vi "Instrument_Setting.vi"(8 "错误输入（无错误）":errorcluster, 9 "id":string[](array[string]), 10 "Get_USB_Resouce":string[](array[string]), 11 "Address Cluster":T1={"SPU"=refnum, "MPM"=[], "Port_Count"=0.0, "MPM_Count"=0.0, "SPU_Resource"=[], "USB_Resource"=[], "MPM_Communicater"="", "MPM_Count"=0.0, "MPM_Address"=[], "MPM_Portnumber"=[], "SPU_DeviveID"="", "MPM_communcation_method"=[], "TSL_sweepstartwave"=0.0, "TSL_sweepstopwave"=0.0, "TSL_Address"="", "TSL_Communicater"="", "TSL"=refnum, "tsl_communcation_method"=3, "TSL_Portnumber"=0.0} {"tsl_communcation_method" items=["GPIB", "C232C", "TCPIP", "USB"]; "MPM_communcation_method" items=["GPIB", "C232C", "TCPIP", "USB"]}) -> (0 "错误输出":errorcluster, 2 "PowerMonitorType":enum16{"DAQ", "MPM_220", "TSL_LOGG"}(ring), 3 "Address Cluster out":T1={"SPU"=refnum, "MPM"=[], "Port_Count"=0.0, "MPM_Count"=0.0, "SPU_Resource"=[], "USB_Resource"=[], "MPM_Communicater"="", "MPM_Count"=0.0, "MPM_Address"=[], "MPM_Portnumber"=[], "SPU_DeviveID"="", "MPM_communcation_method"=[], "TSL_sweepstartwave"=0.0, "TSL_sweepstopwave"=0.0, "TSL_Address"="", "TSL_Communicater"="", "TSL"=refnum, "tsl_communcation_method"=3, "TSL_Portnumber"=0.0} {"tsl_communcation_method" items=["GPIB", "C232C", "TCPIP", "USB"]; "MPM_communcation_method" items=["GPIB", "C232C", "TCPIP", "USB"]})   [LabVIEW 2017]
doc: "Setting Form"
uses:
  CTL/Address Cluster.ctl
  D:/test/ILSTS/LV_IL/LV_IL_Sample_x86/DLL/InstrumentDLL.dll
  DLL/InstrumentDLL.dll
  Share/PowerMonitorType.vi
panel:
  in  "Product_MPM":enum32{"rdompm210", "rdompm220"}(radio) caption="Product"
  in  "Preformance":enum32{"rb_high_spec", "rb_standard"}(radio)
  out "Boolean":bool=TRUE
  in  "Port_Count":i32
  in  "btnconnect":bool
  in  "cmbSPU_dev":u16(ring) caption="Device"
  in  "IP Address_MPM 2":string caption="IP Address"
  in  "LAN Port_MPM 2":dbl caption="LAN Port"
  in  "GPIB Address_MPM 2":i32 caption="GPIB Address"
  in  "chkmulti_dev":bool
  in  "IP Address_MPM":string caption="IP Address"
  in  "LAN Port_MPM":dbl caption="LAN Port"
  in  "GPIB Address_MPM":i32=14 caption="GPIB Address"
  in  "Communication_MPM":enum32{"rdiGPIB_MPM", "rdiLAN_MPM"}(radio) caption="Communication"
  in  "IP Address_TSL":string caption="IP Address"
  in  "LAN Port_TSL":i32 caption="LAN Port"
  in  "GPIB Address_TSL":i32=1 caption="GPIB Address"
  in  "Usb resouce_TSL":u16(ring) caption="Usb resouce"
  in  "Communication_TSL":T2(radio) caption="Communication"
  in  "Product_TSL":enum32{"rdo550_TSL", "rdo570_TSL"}(radio) caption="Product"
  # "TSL"
  # "MPM"
  # "Device1"
  # "Device2"
  # "SPU"
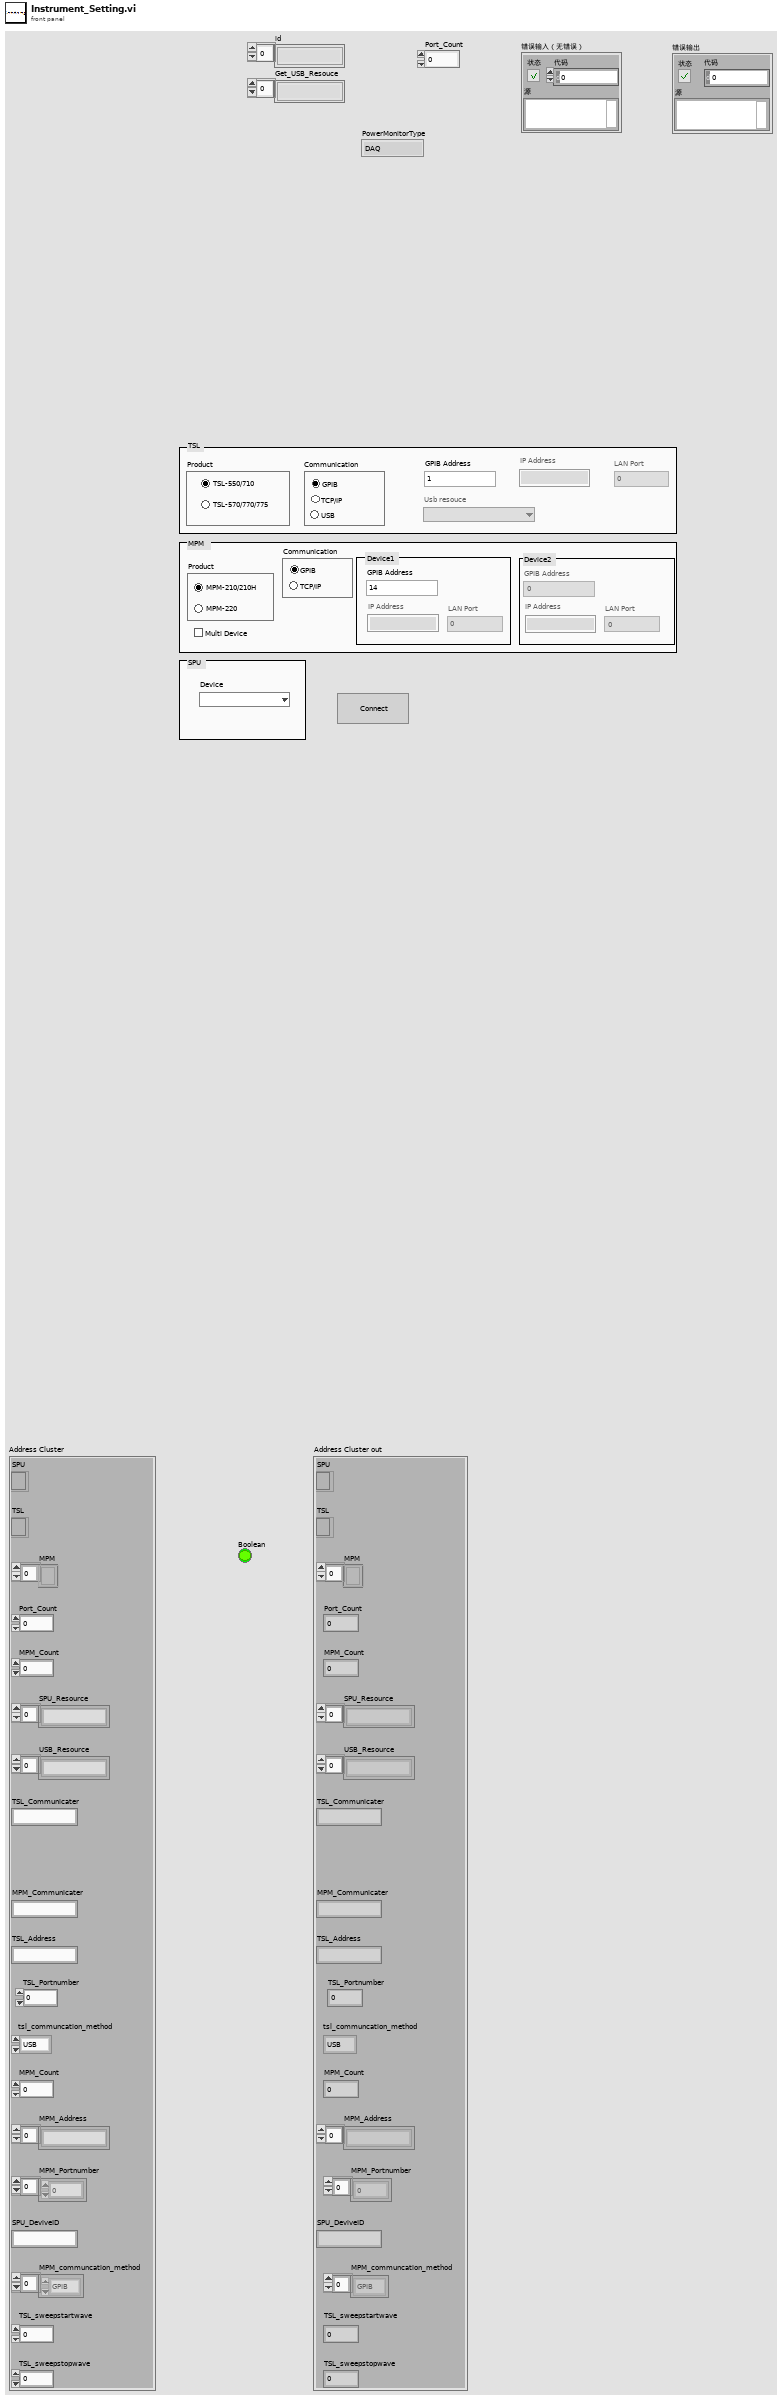
[diagram p1: front panel]
types:
  T1 = typedef "Address Cluster.ctl" = cluster{"SPU":refnum<k24>, "MPM":refnum<k24>[], "Port_Count":dbl, "MPM_Count":dbl, "SPU_Resource":string[], "USB_Resource":string[], "MPM_Communicater":string, "MPM_Count":dbl, "MPM_Address":string[], "MPM_Portnumber":dbl[], "SPU_DeviveID":string, "MPM_communcation_method":i32[], "TSL_sweepstartwave":dbl, "TSL_sweepstopwave":dbl, "TSL_Address":string, "TSL_Communicater":string, "TSL":refnum<k24>, "tsl_communcation_method":i32, "TSL_Portnumber":dbl}
  T2 = enum32{"rdiGPIB_TSL", "rdiLAN_TSL", "rdiUSB_TSL"}
  T3 = enum8{"Enabled", "Disabled", "Disabled and Grayed Out"}
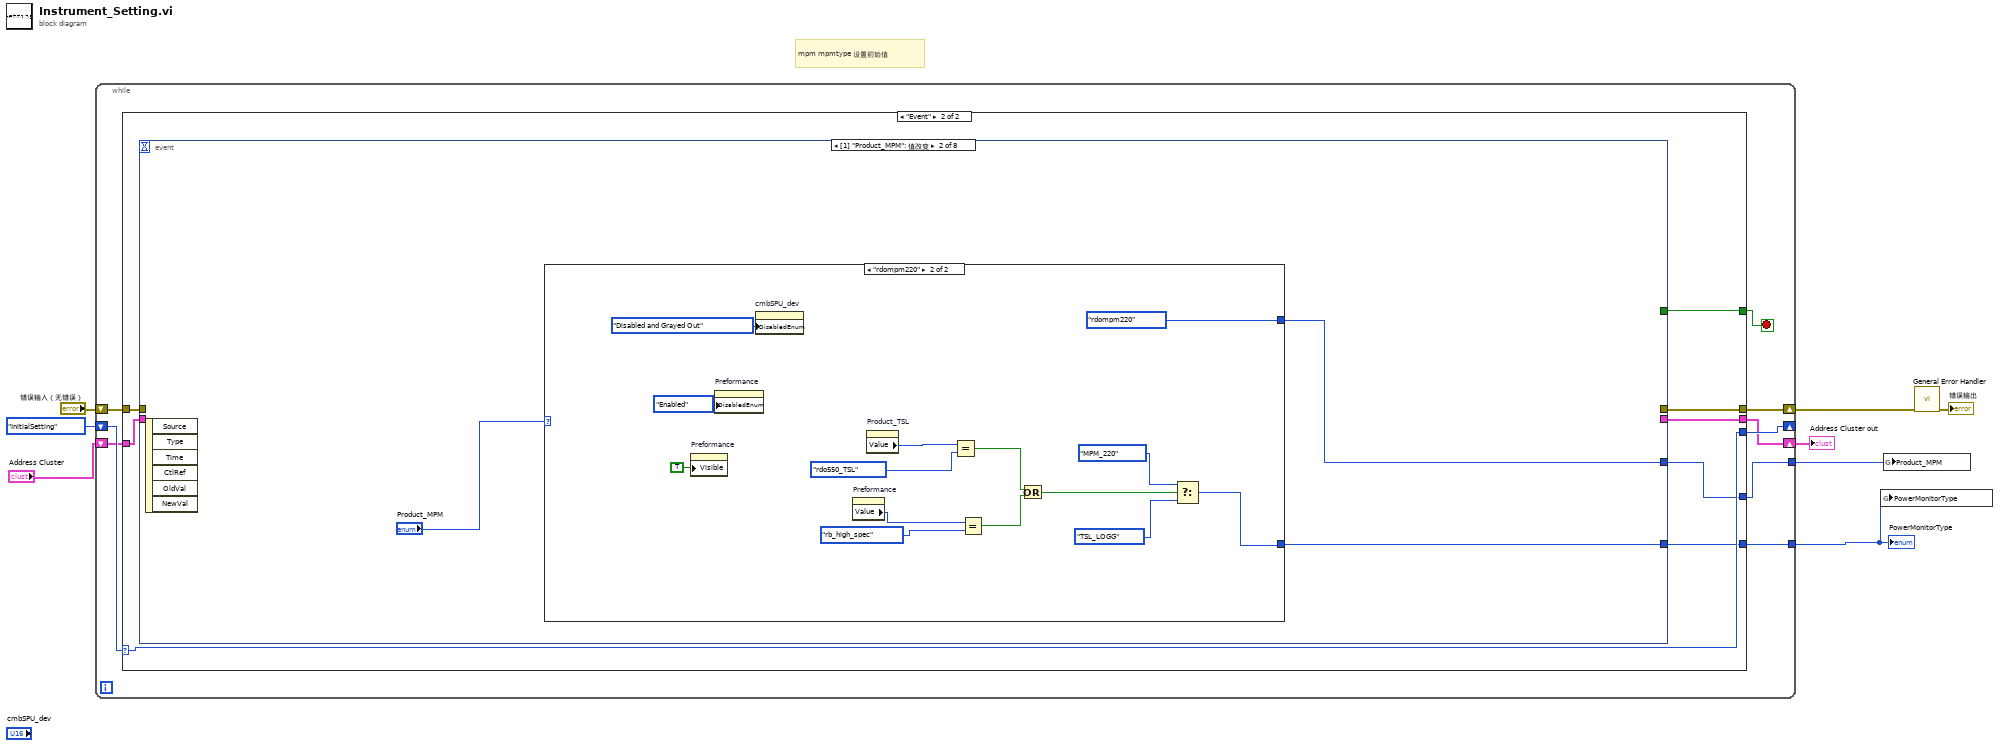
[diagram p0: block diagram]
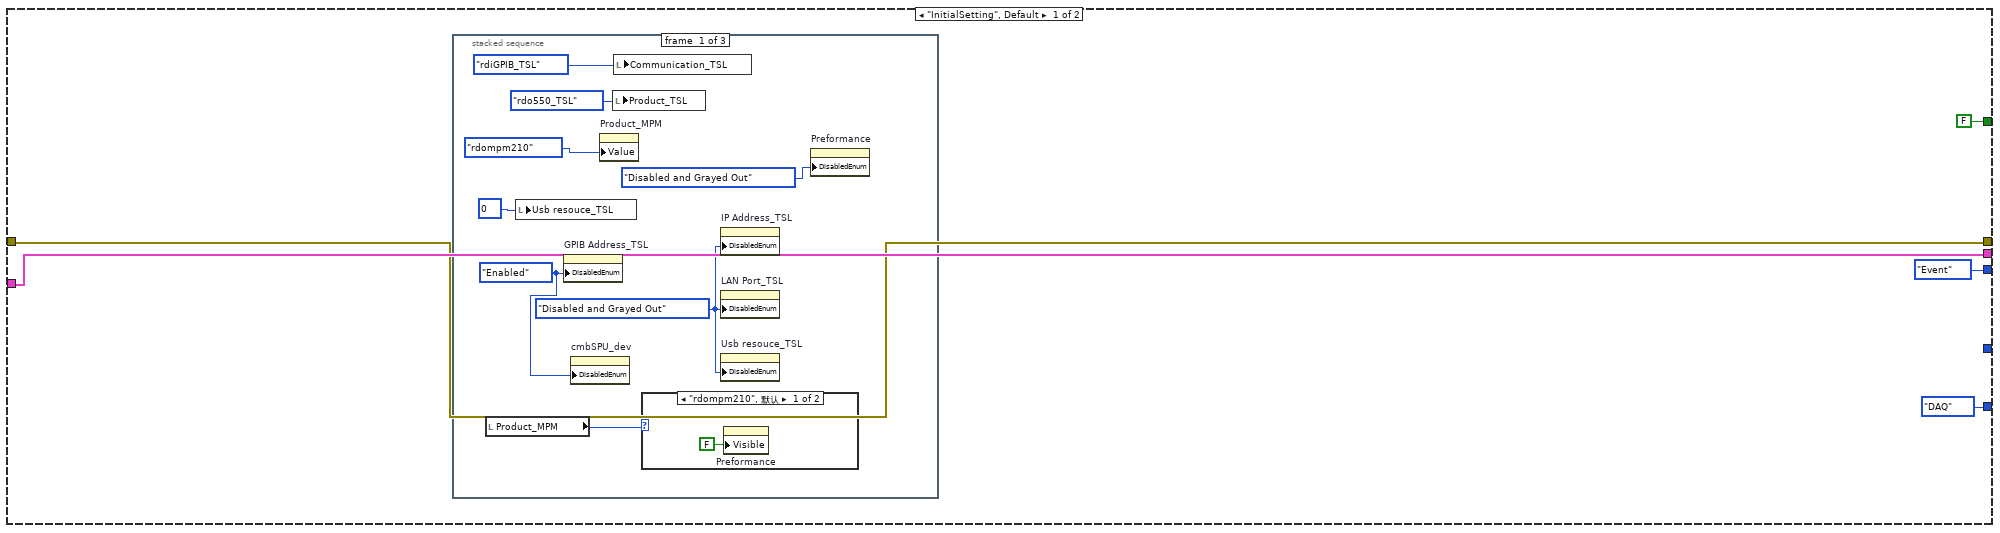
[diagram p2: hidden frame]
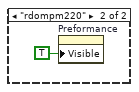
[diagram p3: hidden frame]
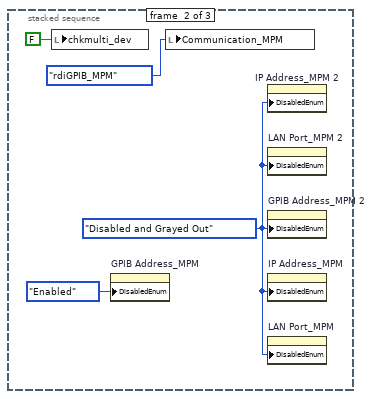
[diagram p4: hidden frame]
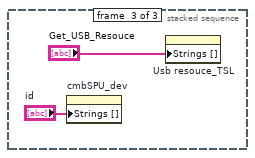
[diagram p5: hidden frame]
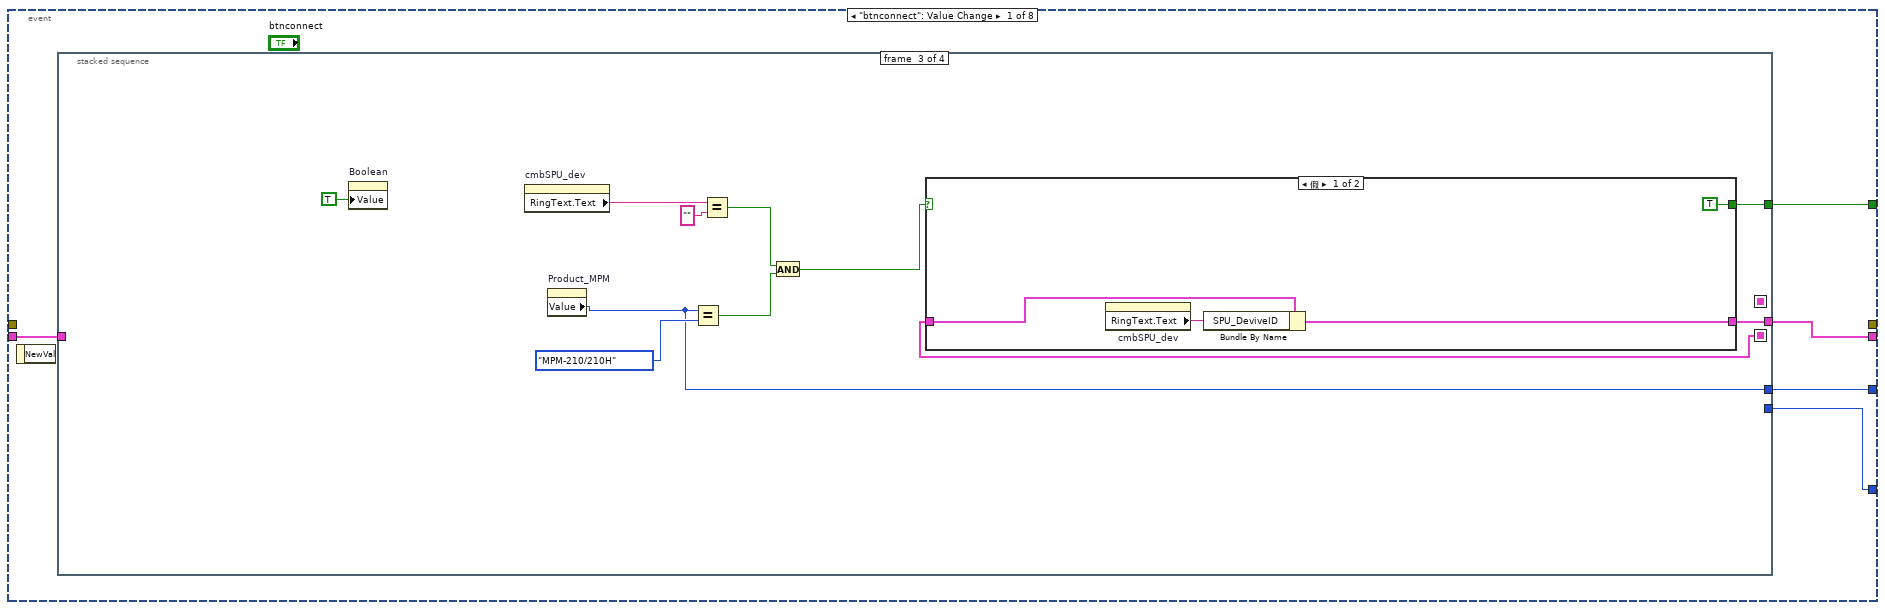
[diagram p6: hidden frame]
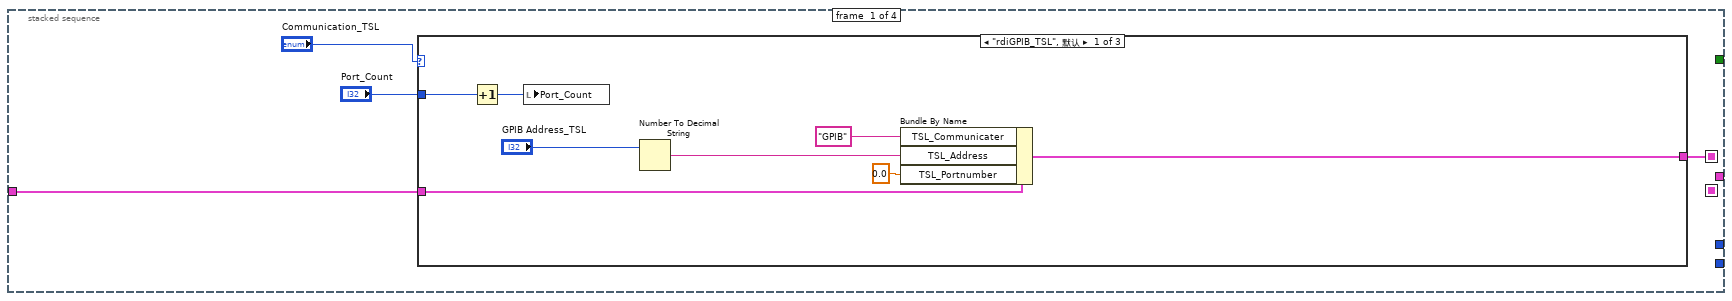
[diagram p7: hidden frame]
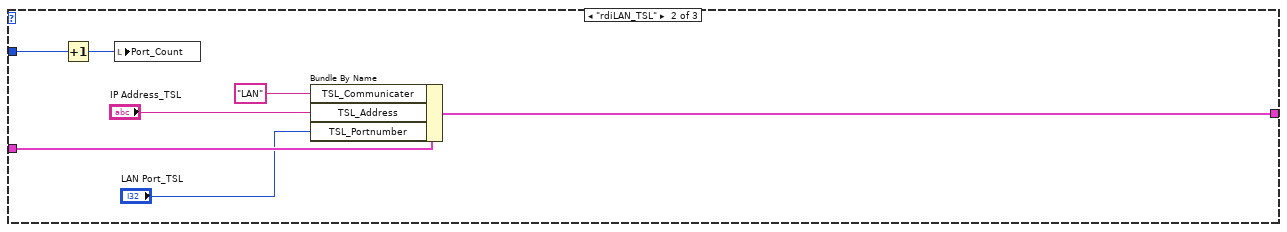
[diagram p8: hidden frame]
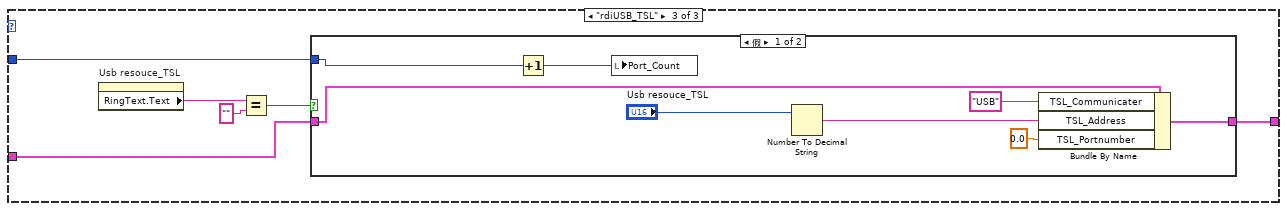
[diagram p9: hidden frame]
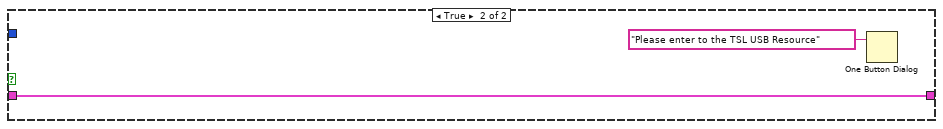
[diagram p10: hidden frame]
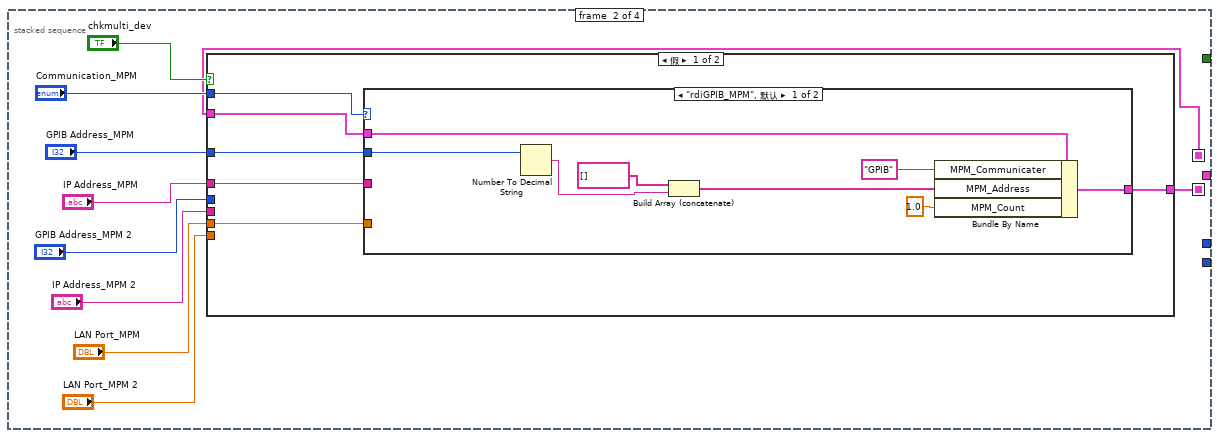
[diagram p11: hidden frame]
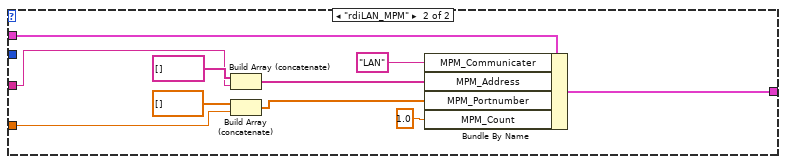
[diagram p12: hidden frame]
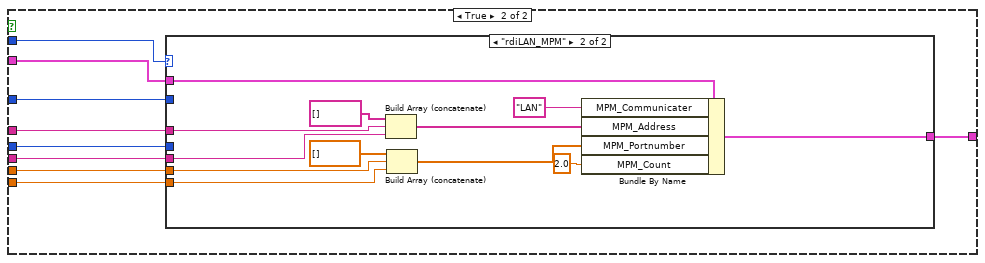
[diagram p13: hidden frame]
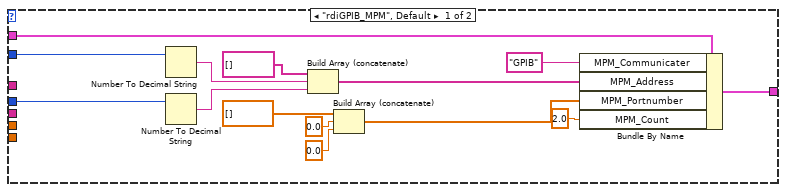
[diagram p14: hidden frame]
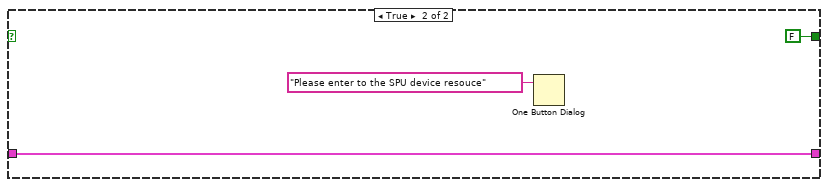
[diagram p15: hidden frame]
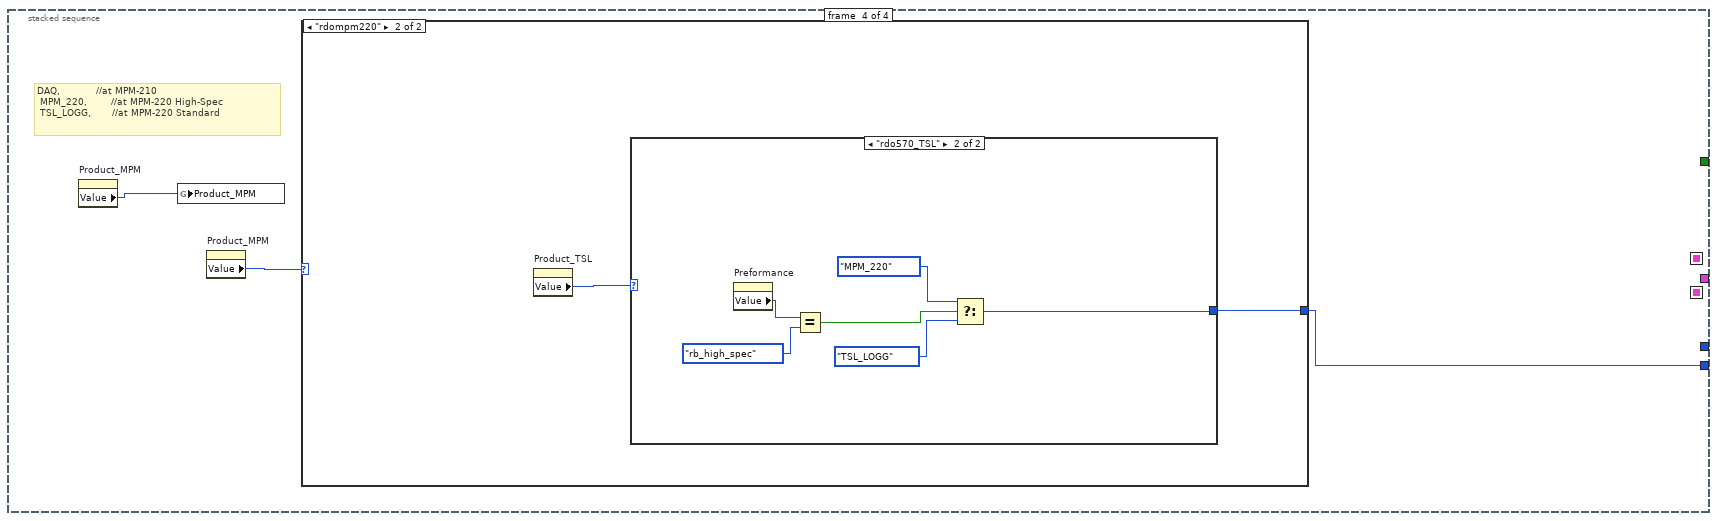
[diagram p16: hidden frame]
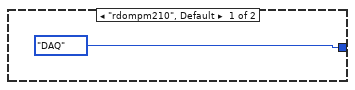
[diagram p17: hidden frame]
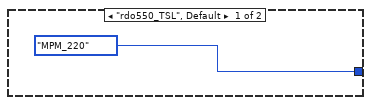
[diagram p18: hidden frame]
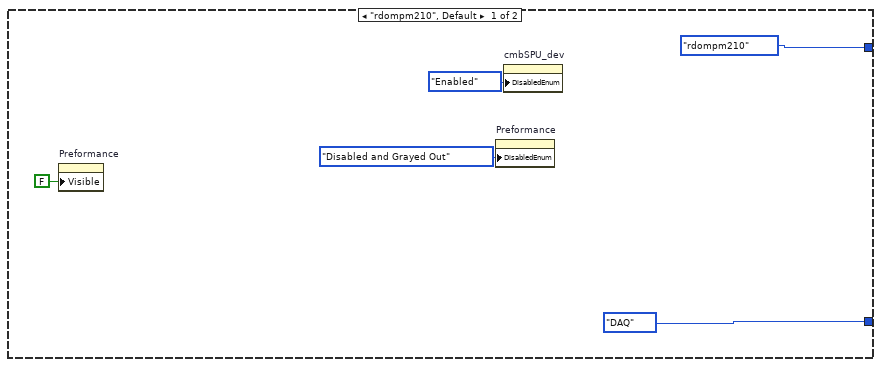
[diagram p19: hidden frame]
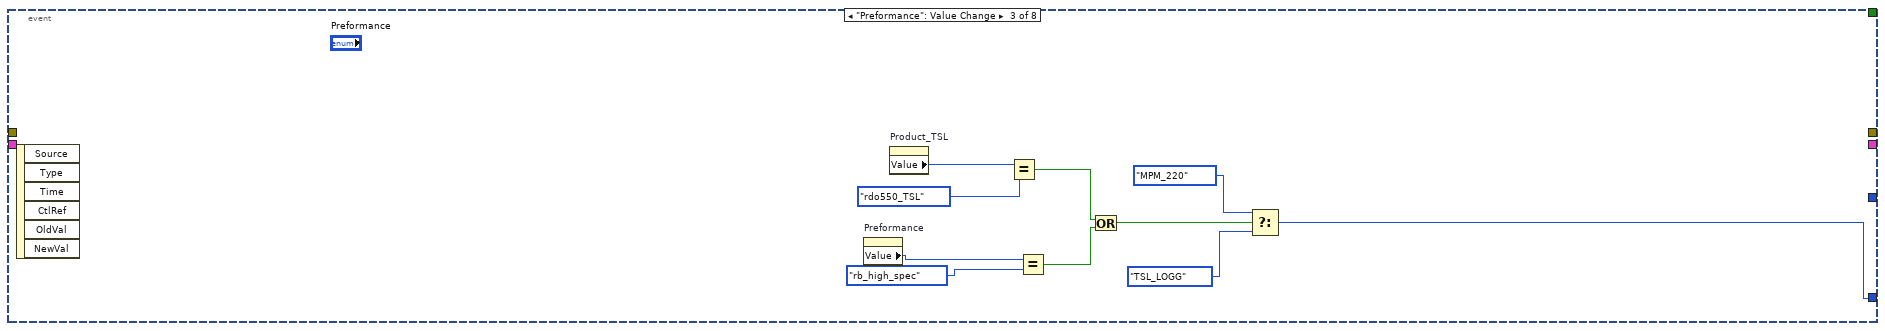
[diagram p20: hidden frame]
diagram:
  # "mpm mpmtype 设置初始值"
  n1 = while {
    shift-right: [w16] -> w6
    shift-left: "错误输入（无错误）" -> [w17]
    shift-right: [w14] -> _
    shift-left: enum16{"InitialSetting", "Event", "Set", "Exit"}."InitialSetting" -> [w15]
    shift-right: [w12] -> w3
    shift-left: "Address Cluster" -> [w13]
    tunnel: [w10] -> w2
    tunnel: [w9] -> w1
    stop <- w11 stop-if-true
    n2 = case shown="\"Event\"" w15 {
      selector: w15 -> [_ w42]
      tunnel: w17 -> [w19 w46]
      tunnel: [w19 w45] -> w16
      tunnel: [FALSE ("status") w41] -> w11
      tunnel: [enum16{"InitialSetting", "Event", "Set", "Exit"}."Event" w42] -> w14
      tunnel: w13 -> [w20 w44]
      tunnel: [w20 w43] -> w12
      tunnel: [enum16{"DAQ", "MPM_220", "TSL_LOGG"}."DAQ" ("PowerMonitorType") w40] -> w10
      tunnel: [_ w39] -> w9
      frame "InitialSetting", Default {
        n3 = stacked-sequence {
          frame #0 {
            w23 = T3."Enabled" ("禁用")
            w29 = T3."Disabled and Grayed Out" ("禁用")
            w30 = u16 0 items=[""] ("Usb resouce_TSL1")
            n4 = local read "Product_MPM"() -> (w25:enum32{"rdompm210", "rdompm220"})
            n5 = local write "Usb resouce_TSL"(w30) -> ()
            n6 = property on="GPIB Address_TSL" class="DigNum (严格)"("DisabledEnum"=w23) -> ()  [unwired: 2 in, 2 out]
            n7 = property on="cmbSPU_dev" class="Ring (严格)"("DisabledEnum"=w23) -> ()  [unwired: 2 in, 2 out]
            n8 = property on="Product_MPM" class="RadioBtnsControl (严格)"("Value"=enum32{"rdompm210", "rdompm220"}."rdompm210" ("Product_MPM")) -> ()  [unwired: 2 in, 2 out]
            n9 = local write "Product_TSL"(enum32{"rdo550_TSL", "rdo570_TSL"}."rdo550_TSL" ("Product_TSL")) -> ()
            n10 = local write "Communication_TSL"(T2."rdiGPIB_TSL" ("Communication_TSL")) -> ()
            n11 = case shown="\"rdompm210\", 默认" w25 {
              frame "rdompm210", Default {
                n12 = property on="Preformance" class="RadioBtnsControl (严格)"("Visible"=FALSE) -> ()  [unwired: 2 in, 2 out]
              }
              frame "rdompm220" {
                n13 = property on="Preformance" class="RadioBtnsControl (严格)"("Visible"=TRUE) -> ()  [unwired: 2 in, 2 out]
              }
            }
            n14 = property on="IP Address_TSL" class="Str"("DisabledEnum"=w29) -> ()  [unwired: 2 in, 2 out]
            n15 = property on="LAN Port_TSL" class="DigNum (严格)"("DisabledEnum"=w29) -> ()  [unwired: 2 in, 2 out]
            n16 = property on="Usb resouce_TSL" class="Ring (严格)"("DisabledEnum"=w29) -> ()  [unwired: 2 in, 2 out]
            n17 = property on="Preformance" class="RadioBtnsControl (严格)"("DisabledEnum"=T3."Disabled and Grayed Out" ("Disabled")) -> ()  [unwired: 2 in, 2 out]
          }
          frame #1 {
            w33 = T3."Disabled and Grayed Out" ("禁用")
            n18 = local write "chkmulti_dev"(FALSE ("chkmulti_dev")) -> ()
            n19 = property on="GPIB Address_MPM" class="DigNum (严格)"("DisabledEnum"=T3."Enabled" ("禁用")) -> ()  [unwired: 2 in, 2 out]
            n20 = local write "Communication_MPM"(enum32{"rdiGPIB_MPM", "rdiLAN_MPM"}."rdiGPIB_MPM" ("Communication_MPM")) -> ()
            n21 = property on="IP Address_MPM 2" class="Str"("DisabledEnum"=w33) -> ()  [unwired: 2 in, 2 out]
            n22 = property on="LAN Port_MPM 2" class="DigNum (严格)"("DisabledEnum"=w33) -> ()  [unwired: 2 in, 2 out]
            n23 = property on="GPIB Address_MPM 2" class="DigNum (严格)"("DisabledEnum"=w33) -> ()  [unwired: 2 in, 2 out]
            n24 = property on="IP Address_MPM" class="Str"("DisabledEnum"=w33) -> ()  [unwired: 2 in, 2 out]
            n25 = property on="LAN Port_MPM" class="DigNum (严格)"("DisabledEnum"=w33) -> ()  [unwired: 2 in, 2 out]
          }
          frame #2 {
            n26 = property on="cmbSPU_dev" class="Ring (严格)"("Strings []"="id") -> ()  [unwired: 2 in, 2 out]
            n27 = property on="Usb resouce_TSL" class="Ring (严格)"("Strings []"="Get_USB_Resouce") -> ()  [unwired: 2 in, 2 out]
          }
        }
      }
      frame "Event" {
        n28 = event shown="[1] \"Product_MPM\": 值改变" {
          selector: _ -> [_ _ _ _ _ _ _ _]
          dyn-events: _ -> [_ _ _ _ _ _ _ _]
          timeout: _ -> [_ _ _ _ _ _ _ _]
          tunnel: w46 -> [_ _ _ w220 w233 w242 w251 _]
          tunnel: [_ _ _ w220 w233 w242 w251 _] -> w45
          tunnel: w44 -> [w51 _ _ _ _ _ _ w266]
          tunnel: [w50 _ _ _ _ _ _ w266] -> w43
          tunnel: [w49 _ _ FALSE ("y") FALSE ("y") FALSE ("y") FALSE ("y") TRUE ("y")] -> w41
          tunnel: [w48 w188 w210 _ _ _ _ _] -> w40
          tunnel: [w47 w187 _ _ _ _ _ _] -> w39
          event "btnconnect": Value Change {
            n29 = event-data() -> ()  [unwired: 1 in, 1 out]
            n30 = stacked-sequence {
              seq-local: [w54 _ _ _] -> [_ w87 _ _]
              seq-local: [_ w88 _ _] -> [_ _ w162 _]
              tunnel: w51 -> [w55 _ _ _]
              tunnel: [_ _ w164 _] -> w50
              tunnel: [_ _ w163 _] -> w49
              tunnel: [_ _ _ w175] -> w48
              tunnel: [_ _ w156 _] -> w47
              frame #0 {
                n31 = case shown="\"rdiGPIB_TSL\", 默认" "Communication_TSL" {
                  tunnel: "Port_Count" -> [w59 w68 w73]
                  tunnel: w55 -> [w62 w70 w72]
                  tunnel: [w61 w69 w71] -> w54
                  frame "rdiGPIB_TSL", Default {
                    n32 = Increment(x=w59) -> (x+1=w60:i32)
                    n33 = local write "Port_Count"(w60) -> ()
                    n34 = Number To Decimal String(number="GPIB Address_TSL") -> (decimal integer string=w57:string)  [unwired: 1 in]
                    n35 = Bundle By Name(cluster=w62, "TSL_Communicater"="GPIB" ("新元素/子数组"), "TSL_Address"=w57, "TSL_Portnumber"=0.0 ("新元素/子数组")) -> (w61:T1)
                  }
                  frame "rdiLAN_TSL" {
                    n36 = Increment(x=w68) -> (x+1=w67:i32)
                    n37 = local write "Port_Count"(w67) -> ()
                    n38 = Bundle By Name(cluster=w70, "TSL_Communicater"="LAN" ("新元素/子数组"), "TSL_Address"="IP Address_TSL", "TSL_Portnumber"="LAN Port_TSL") -> (w69:T1)
                  }
                  frame "rdiUSB_TSL" {
                    n39 = property on="Usb resouce_TSL" class="Ring (严格)"() -> ("RingText.Text"=w76:string)  [unwired: 2 in, 2 out]
                    n40 = Equal?(x=w76, y="") -> (x = y?=w74:bool)
                    n41 = case shown="假" w74 {
                      tunnel: w73 -> [w80 _]
                      tunnel: w72 -> [w83 w85]
                      tunnel: [w82 w85] -> w71
                      frame False {
                        n42 = Increment(x=w80) -> (x+1=w81:i32)
                        n43 = local write "Port_Count"(w81) -> ()
                        n44 = Number To Decimal String(number="Usb resouce_TSL") -> (decimal integer string=w78:string)  [unwired: 1 in]
                        n45 = Bundle By Name(cluster=w83, "TSL_Communicater"="USB" ("新元素/子数组"), "TSL_Address"=w78, "TSL_Portnumber"=0.0 ("新元素/子数组")) -> (w82:T1)
                      }
                      frame True {
                        n46 = One Button Dialog(message="Please enter to the TSL USB Resource" ("消息")) -> ()  [unwired: 1 in, 1 out]
                      }
                    }
                  }
                }
              }
              frame #1 {
                n47 = case shown="假" "chkmulti_dev" {
                  tunnel: w87 -> [w98 w129]
                  tunnel: "Communication_MPM" -> [w102 w128]
                  tunnel: [w99 w127] -> w88
                  tunnel: "GPIB Address_MPM 2" -> [_ w126]
                  tunnel: "GPIB Address_MPM" -> [w97 w125]
                  tunnel: "LAN Port_MPM 2" -> [_ w124]
                  tunnel: "LAN Port_MPM" -> [w101 w123]
                  tunnel: "IP Address_MPM 2" -> [_ w122]
                  tunnel: "IP Address_MPM" -> [w100 w121]
                  frame False {
                    n48 = case shown="\"rdiGPIB_MPM\", 默认" w102 {
                      tunnel: w101 -> [_ w117]
                      tunnel: w100 -> [_ w114]
                      tunnel: [w107 w112] -> w99
                      tunnel: w98 -> [w108 w111]
                      tunnel: w97 -> [w104 _]
                      frame "rdiGPIB_MPM", Default {
                        n49 = Number To Decimal String(number=w104) -> (decimal integer string=w105:string)  [unwired: 1 in]
                        n50 = Build Array (concatenate)(string[] [] ("MPM_Address"), w105) -> (w103:string[])
                        n51 = Bundle By Name(cluster=w108, "MPM_Communicater"="GPIB", "MPM_Address"=w103, "MPM_Count"=1.0) -> (w107:T1)
                      }
                      frame "rdiLAN_MPM" {
                        n52 = Build Array (concatenate)(string[] [] ("MPM_Address"), w114) -> (w113:string[])
                        n53 = Build Array (concatenate)(dbl[] [] ("MPM_Portnumber"), w117) -> (w116:dbl[])
                        n54 = Bundle By Name(cluster=w111, "MPM_Communicater"="LAN", "MPM_Address"=w113, "MPM_Portnumber"=w116, "MPM_Count"=1.0) -> (w112:T1)
                      }
                    }
                  }
                  frame True {
                    n55 = case shown="\"rdiLAN_MPM\"" w128 {
                      tunnel: w129 -> [w137 w155]
                      tunnel: [w132 w144] -> w127
                      tunnel: w126 -> [w131 _]
                      tunnel: w125 -> [w130 _]
                      tunnel: w124 -> [_ w148]
                      tunnel: w123 -> [_ w147]
                      tunnel: w122 -> [_ w146]
                      tunnel: w121 -> [_ w145]
                      frame "rdiGPIB_MPM", Default {
                        n56 = Number To Decimal String(number=w130) -> (decimal integer string=w140:string)  [unwired: 1 in]
                        n57 = Number To Decimal String(number=w131) -> (decimal integer string=w139:string)  [unwired: 1 in]
                        n58 = Build Array (concatenate)(string[] [] ("MPM_Address"), w140, w139) -> (w138:string[])
                        n59 = Build Array (concatenate)(dbl[] [] ("MPM_Portnumber"), 0.0 ("新元素/子数组"), 0.0 ("新元素/子数组")) -> (w133:dbl[])
                        n60 = Bundle By Name(cluster=w137, "MPM_Communicater"="GPIB", "MPM_Address"=w138, "MPM_Portnumber"=w133, "MPM_Count"=2.0) -> (w132:T1)
                      }
                      frame "rdiLAN_MPM" {
                        n61 = Build Array (concatenate)(string[] [] ("MPM_Address"), w145, w146) -> (w151:string[])
                        n62 = Build Array (concatenate)(dbl[] [] ("MPM_Portnumber"), w147, w148) -> (w149:dbl[])
                        n63 = Bundle By Name(cluster=w155, "MPM_Communicater"="LAN", "MPM_Address"=w151, "MPM_Portnumber"=w149, "MPM_Count"=2.0) -> (w144:T1)
                      }
                    }
                  }
                }
              }
              frame #2 {
                n64 = property on="Boolean" class="Bool (严格)"("Value"=TRUE ("Boolean")) -> ()  [unwired: 2 in, 2 out]
                n65 = property on="cmbSPU_dev" class="Ring (严格)"() -> ("RingText.Text"=w166:string)  [unwired: 2 in, 2 out]
                n66 = property on="Product_MPM" class="RadioBtnsControl (严格)"() -> ("Value"=w156:enum32{"rdompm210", "rdompm220"})  [unwired: 2 in, 2 out]
                n67 = Equal?(x=w156, y=enum32{"MPM-210/210H", "MPM-220"}."MPM-210/210H") -> (x = y?=w159:bool)
                n68 = Equal?(x=w166, y="") -> (x = y?=w160:bool)
                n69 = And(x=w160, y=w159) -> (x .and. y?=w158:bool)
                n70 = case shown="假" w158 {
                  tunnel: w162 -> [w170 w172]
                  tunnel: [w169 w172] -> w164
                  tunnel: [TRUE ("y") FALSE ("y")] -> w163
                  frame False {
                    n71 = property on="cmbSPU_dev" class="Ring (严格)"() -> ("RingText.Text"=w168:string)  [unwired: 2 in, 2 out]
                    n72 = Bundle By Name(cluster=w170, "SPU_DeviveID"=w168) -> (w169:T1)
                  }
                  frame True {
                    n73 = One Button Dialog(message="Please enter to the SPU device resouce" ("消息")) -> ()  [unwired: 1 in, 1 out]
                  }
                }
              }
              frame #3 {
                # "DAQ,            //at MPM-210\n MPM_220,        //at MPM-220 High-Spec\n TSL_LOGG,       //at MPM-220 Standard"
                n74 = property on="Product_MPM" class="RadioBtnsControl (严格)"() -> ("Value"=w174:enum32{"rdompm210", "rdompm220"})  [unwired: 2 in, 2 out]
                n75 = global write "PowerMonitorType.vi" "Product_MPM"(w174) -> ()
                n76 = property on="Product_MPM" class="RadioBtnsControl (严格)"() -> ("Value"=w176:enum32{"rdompm210", "rdompm220"})  [unwired: 2 in, 2 out]
                n77 = case shown="\"rdompm220\"" w176 {
                  tunnel: [enum16{"DAQ", "MPM_220", "TSL_LOGG"}."DAQ" ("PowerMonitorType") w179] -> w175
                  frame "rdompm210", Default {
                  }
                  frame "rdompm220" {
                    n78 = property on="Product_TSL" class="RadioBtnsControl (严格)"() -> ("Value"=w178:enum32{"rdo550_TSL", "rdo570_TSL"})  [unwired: 2 in, 2 out]
                    n79 = case shown="\"rdo570_TSL\"" w178 {
                      tunnel: [enum16{"DAQ", "MPM_220", "TSL_LOGG"}."MPM_220" ("PowerMonitorType") w182] -> w179
                      frame "rdo550_TSL", Default {
                      }
                      frame "rdo570_TSL" {
                        n80 = property on="Preformance" class="RadioBtnsControl (严格)"() -> ("Value"=w184:enum32{"rb_high_spec", "rb_standard"})  [unwired: 2 in, 2 out]
                        n81 = Equal?(x=w184, y=enum32{"rb_high_spec", "rb_standard"}."rb_high_spec") -> (x = y?=w183:bool)
                        n82 = Select(t=enum16{"DAQ", "MPM_220", "TSL_LOGG"}."MPM_220" ("PowerMonitorType"), s=w183, f=enum16{"DAQ", "MPM_220", "TSL_LOGG"}."TSL_LOGG") -> (s? t:f=w182:enum16{"DAQ", "MPM_220", "TSL_LOGG"})
                      }
                    }
                  }
                }
              }
            }
          }
          event "Product_MPM": Value Change {
            n83 = event-data() -> ()  [unwired: 1 in, 6 out]
            n84 = case shown="\"rdompm220\"" "Product_MPM" {
              tunnel: [enum16{"DAQ", "MPM_220", "TSL_LOGG"}."DAQ" ("PowerMonitorType") w197] -> w188
              tunnel: [enum32{"rdompm210", "rdompm220"}."rdompm210" ("Product_MPM") enum32{"rdompm210", "rdompm220"}."rdompm220" ("Product_MPM")] -> w187
              frame "rdompm210", Default {
                n85 = property on="Preformance" class="RadioBtnsControl (严格)"("Visible"=FALSE) -> ()  [unwired: 2 in, 2 out]
                n86 = property on="Preformance" class="RadioBtnsControl (严格)"("DisabledEnum"=T3."Disabled and Grayed Out" ("Disabled")) -> ()  [unwired: 2 in, 2 out]
                n87 = property on="cmbSPU_dev" class="Ring (严格)"("DisabledEnum"=T3."Enabled" ("Disabled")) -> ()  [unwired: 2 in, 2 out]
              }
              frame "rdompm220" {
                n88 = property on="Preformance" class="RadioBtnsControl (严格)"("Visible"=TRUE) -> ()  [unwired: 2 in, 2 out]
                n89 = property on="Preformance" class="RadioBtnsControl (严格)"("DisabledEnum"=T3."Enabled" ("Disabled")) -> ()  [unwired: 2 in, 2 out]
                n90 = property on="cmbSPU_dev" class="Ring (严格)"("DisabledEnum"=T3."Disabled and Grayed Out" ("Disabled")) -> ()  [unwired: 2 in, 2 out]
                n91 = property on="Preformance" class="RadioBtnsControl (严格)"() -> ("Value"=w202:enum32{"rb_high_spec", "rb_standard"})  [unwired: 2 in, 2 out]
                n92 = property on="Product_TSL" class="RadioBtnsControl (严格)"() -> ("Value"=w205:enum32{"rdo550_TSL", "rdo570_TSL"})  [unwired: 2 in, 2 out]
                n93 = Equal?(x=w205, y=enum32{"rdo550_TSL", "rdo570_TSL"}."rdo550_TSL") -> (x = y?=w200:bool)
                n94 = Equal?(x=w202, y=enum32{"rb_high_spec", "rb_standard"}."rb_high_spec") -> (x = y?=w199:bool)
                n95 = Or(x=w200, y=w199) -> (x .or. y?=w198:bool)
                n96 = Select(t=enum16{"DAQ", "MPM_220", "TSL_LOGG"}."MPM_220", s=w198, f=enum16{"DAQ", "MPM_220", "TSL_LOGG"}."TSL_LOGG" ("PowerMonitorType")) -> (s? t:f=w197:enum16{"DAQ", "MPM_220", "TSL_LOGG"})
              }
            }
          }
          event "Preformance": Value Change {
            n97 = event-data() -> ()  [unwired: 1 in, 6 out]
            n98 = property on="Preformance" class="RadioBtnsControl (严格)"() -> ("Value"=w215:enum32{"rb_high_spec", "rb_standard"})  [unwired: 2 in, 2 out]
            n99 = property on="Product_TSL" class="RadioBtnsControl (严格)"() -> ("Value"=w214:enum32{"rdo550_TSL", "rdo570_TSL"})  [unwired: 2 in, 2 out]
            n100 = Equal?(x=w214, y=enum32{"rdo550_TSL", "rdo570_TSL"}."rdo550_TSL") -> (x = y?=w216:bool)
            n101 = Equal?(x=w215, y=enum32{"rb_high_spec", "rb_standard"}."rb_high_spec") -> (x = y?=w217:bool)
            n102 = Or(x=w216, y=w217) -> (x .or. y?=w218:bool)
            n103 = Select(t=enum16{"DAQ", "MPM_220", "TSL_LOGG"}."MPM_220", s=w218, f=enum16{"DAQ", "MPM_220", "TSL_LOGG"}."TSL_LOGG" ("PowerMonitorType")) -> (s? t:f=w210:enum16{"DAQ", "MPM_220", "TSL_LOGG"})
          }
          event "Product_TSL": Value Change {
            n104 = event-data() -> ()  [unwired: 1 in, 1 out]
            n105 = flat-sequence {
              tunnel: [w223] -> w219
              tunnel: w220 -> [w223]
              frame #0 {
                n106 = property on="Preformance" class="RadioBtnsControl (严格)"("DisabledEnum"=T3."Enabled" ("Disabled")) -> ()  [unwired: 2 in, 2 out]
              }
            }
            n107 = case shown="\"rdo550_TSL\", 默认" "Product_TSL" {
              tunnel: w219 -> [_ _]
              frame "rdo550_TSL", Default {
                w229 = T3."Disabled and Grayed Out" ("禁用")
                # "'TSL-550/710\n' There can control only GPIB"
                n108 = property on="Product_MPM" class="RadioBtnsControl (严格)"() -> ("Value"=w227:enum32{"rdompm210", "rdompm220"})  [unwired: 2 in, 2 out]
                n109 = property on="rdiGPIB_TSL" class="Bool (严格)"("Value"=TRUE ("键选中")) -> ()  [unwired: 2 in, 2 out]
                n110 = Equal?(x=w227, y=enum32{"MPM-210/210H", "MPM-220"}."MPM-220") -> (x = y?=w225:bool)
                n111 = property on="rdiLAN_TSL" class="Bool (严格)"("DisabledEnum"=w229) -> ()  [unwired: 2 in, 2 out]
                n112 = property on="rdiUSB_TSL" class="Bool (严格)"("DisabledEnum"=w229) -> ()  [unwired: 2 in, 2 out]
                n113 = case shown="真" w225 {
                  frame False {
                  }
                  frame True {
                    n114 = property on="Preformance" class="RadioBtnsControl (严格)"("Value"=enum32{"rb_high_spec", "rb_standard"}."rb_high_spec" ("Preformance")) -> ()  [unwired: 2 in, 2 out]
                    n115 = property on="Preformance" class="RadioBtnsControl (严格)"("DisabledEnum"=T3."Disabled and Grayed Out" ("t")) -> ()  [unwired: 2 in, 2 out]
                  }
                }
              }
              frame "rdo570_TSL" {
                w232 = T3."Enabled" ("禁用")
                # "TSL-570"
                n116 = property on="rdiLAN_TSL" class="Bool (严格)"("DisabledEnum"=w232) -> ()  [unwired: 2 in, 2 out]
                n117 = property on="rdiUSB_TSL" class="Bool (严格)"("DisabledEnum"=w232) -> ()  [unwired: 2 in, 2 out]
              }
            }
          }
          event "Communication_TSL": Value Change {
            n118 = event-data() -> ()  [unwired: 1 in, 1 out]
            n119 = local read "Communication_TSL"() -> (w235:T2)
            n120 = case shown="\"rdiLAN_TSL\"" w235 {
              frame "rdiLAN_TSL" {
                w236 = T3."Enabled" ("禁用")
                w237 = T3."Disabled and Grayed Out" ("禁用")
                # "TSL Control TCP/IP"
                n121 = property on="IP Address_TSL" class="Str"("DisabledEnum"=w236) -> ()  [unwired: 2 in, 2 out]
                n122 = property on="LAN Port_TSL" class="DigNum (严格)"("DisabledEnum"=w236) -> ()  [unwired: 2 in, 2 out]
                n123 = property on="Usb resouce_TSL" class="Ring (严格)"("DisabledEnum"=w237) -> ()  [unwired: 2 in, 2 out]
                n124 = property on="GPIB Address_TSL" class="DigNum (严格)"("DisabledEnum"=w237) -> ()  [unwired: 2 in, 2 out]
              }
              frame "rdiGPIB_TSL", Default {
                w238 = T3."Disabled and Grayed Out" ("禁用")
                # "TSL Control GPIB"
                n125 = property on="GPIB Address_TSL" class="DigNum (严格)"("DisabledEnum"=T3."Enabled" ("禁用")) -> ()  [unwired: 2 in, 2 out]
                n126 = property on="Usb resouce_TSL" class="Ring (严格)"("DisabledEnum"=w238) -> ()  [unwired: 2 in, 2 out]
                n127 = property on="LAN Port_TSL" class="DigNum (严格)"("DisabledEnum"=w238) -> ()  [unwired: 2 in, 2 out]
                n128 = property on="IP Address_TSL" class="Str"("DisabledEnum"=w238) -> ()  [unwired: 2 in, 2 out]
              }
              frame "rdiUSB_TSL" {
                w240 = T3."Disabled and Grayed Out" ("禁用")
                # "TSL Control USB"
                n129 = property on="Usb resouce_TSL" class="Ring (严格)"("DisabledEnum"=T3."Enabled" ("禁用")) -> ()  [unwired: 2 in, 2 out]
                n130 = property on="GPIB Address_TSL" class="DigNum (严格)"("DisabledEnum"=w240) -> ()  [unwired: 2 in, 2 out]
                n131 = property on="LAN Port_TSL" class="DigNum (严格)"("DisabledEnum"=w240) -> ()  [unwired: 2 in, 2 out]
                n132 = property on="IP Address_TSL" class="Str"("DisabledEnum"=w240) -> ()  [unwired: 2 in, 2 out]
              }
            }
          }
          event "chkmulti_dev": Value Change {
            n133 = event-data() -> ()  [unwired: 1 in, 1 out]
            n134 = local read "chkmulti_dev"() -> (w244:bool)
            n135 = case shown="真" w244 {
              frame False {
                w245 = T3."Disabled and Grayed Out" ("禁用")
                n136 = property on="LAN Port_MPM 2" class="DigNum (严格)"("DisabledEnum"=w245) -> ()  [unwired: 2 in, 2 out]
                n137 = property on="IP Address_MPM 2" class="Str"("DisabledEnum"=w245) -> ()  [unwired: 2 in, 2 out]
                n138 = property on="GPIB Address_MPM 2" class="DigNum (严格)"("DisabledEnum"=w245) -> ()  [unwired: 2 in, 2 out]
              }
              frame True {
                n139 = local read "Communication_MPM"() -> (w246:enum32{"rdiGPIB_MPM", "rdiLAN_MPM"})
                n140 = case shown="\"rdiLAN_MPM\"" w246 {
                  frame "rdiLAN_MPM" {
                    w247 = T3."Enabled" ("禁用")
                    n141 = property on="LAN Port_MPM 2" class="DigNum (严格)"("DisabledEnum"=w247) -> ()  [unwired: 2 in, 2 out]
                    n142 = property on="IP Address_MPM 2" class="Str"("DisabledEnum"=w247) -> ()  [unwired: 2 in, 2 out]
                    n143 = property on="GPIB Address_MPM 2" class="DigNum (严格)"("DisabledEnum"=T3."Disabled and Grayed Out" ("禁用")) -> ()  [unwired: 2 in, 2 out]
                  }
                  frame "rdiGPIB_MPM", Default {
                    w249 = T3."Disabled and Grayed Out" ("禁用")
                    n144 = property on="GPIB Address_MPM 2" class="DigNum (严格)"("DisabledEnum"=T3."Enabled" ("禁用")) -> ()  [unwired: 2 in, 2 out]
                    n145 = property on="IP Address_MPM 2" class="Str"("DisabledEnum"=w249) -> ()  [unwired: 2 in, 2 out]
                    n146 = property on="LAN Port_MPM 2" class="DigNum (严格)"("DisabledEnum"=w249) -> ()  [unwired: 2 in, 2 out]
                  }
                }
              }
            }
          }
          event "Communication_MPM": Value Change {
            n147 = event-data() -> ()  [unwired: 1 in, 1 out]
            n148 = local read "Communication_MPM"() -> (w253:enum32{"rdiGPIB_MPM", "rdiLAN_MPM"})
            n149 = case shown="\"rdiGPIB_MPM\", 默认" w253 {
              frame "rdiLAN_MPM" {
                n150 = local read "chkmulti_dev"() -> (w254:bool)
                n151 = case shown="真" w254 {
                  frame True {
                    w255 = T3."Disabled and Grayed Out" ("禁用")
                    w256 = T3."Enabled" ("禁用")
                    n152 = property on="IP Address_MPM" class="Str"("DisabledEnum"=w256) -> ()  [unwired: 2 in, 2 out]
                    n153 = property on="LAN Port_MPM" class="DigNum (严格)"("DisabledEnum"=w256) -> ()  [unwired: 2 in, 2 out]
                    n154 = property on="LAN Port_MPM 2" class="DigNum (严格)"("DisabledEnum"=w256) -> ()  [unwired: 2 in, 2 out]
                    n155 = property on="IP Address_MPM 2" class="Str"("DisabledEnum"=w256) -> ()  [unwired: 2 in, 2 out]
                    n156 = property on="GPIB Address_MPM 2" class="DigNum (严格)"("DisabledEnum"=w255) -> ()  [unwired: 2 in, 2 out]
                    n157 = property on="GPIB Address_MPM" class="DigNum (严格)"("DisabledEnum"=w255) -> ()  [unwired: 2 in, 2 out]
                  }
                  frame False {
                    w257 = T3."Disabled and Grayed Out" ("禁用")
                    w258 = T3."Disabled and Grayed Out" ("禁用")
                    w259 = T3."Enabled" ("禁用")
                    n158 = property on="IP Address_MPM" class="Str"("DisabledEnum"=w259) -> ()  [unwired: 2 in, 2 out]
                    n159 = property on="LAN Port_MPM" class="DigNum (严格)"("DisabledEnum"=w259) -> ()  [unwired: 2 in, 2 out]
                    n160 = property on="IP Address_MPM 2" class="Str"("DisabledEnum"=w257) -> ()  [unwired: 2 in, 2 out]
                    n161 = property on="LAN Port_MPM 2" class="DigNum (严格)"("DisabledEnum"=w257) -> ()  [unwired: 2 in, 2 out]
                    n162 = property on="GPIB Address_MPM 2" class="DigNum (严格)"("DisabledEnum"=w258) -> ()  [unwired: 2 in, 2 out]
                    n163 = property on="GPIB Address_MPM" class="DigNum (严格)"("DisabledEnum"=w258) -> ()  [unwired: 2 in, 2 out]
                  }
                }
              }
              frame "rdiGPIB_MPM", Default {
                n164 = local read "chkmulti_dev"() -> (w260:bool)
                n165 = case shown="假" w260 {
                  frame True {
                    w261 = T3."Enabled" ("禁用")
                    w262 = T3."Disabled and Grayed Out" ("禁用")
                    n166 = property on="GPIB Address_MPM" class="DigNum (严格)"("DisabledEnum"=w261) -> ()  [unwired: 2 in, 2 out]
                    n167 = property on="GPIB Address_MPM 2" class="DigNum (严格)"("DisabledEnum"=w261) -> ()  [unwired: 2 in, 2 out]
                    n168 = property on="IP Address_MPM" class="Str"("DisabledEnum"=w262) -> ()  [unwired: 2 in, 2 out]
                    n169 = property on="LAN Port_MPM" class="DigNum (严格)"("DisabledEnum"=w262) -> ()  [unwired: 2 in, 2 out]
                    n170 = property on="IP Address_MPM 2" class="Str"("DisabledEnum"=w262) -> ()  [unwired: 2 in, 2 out]
                    n171 = property on="LAN Port_MPM 2" class="DigNum (严格)"("DisabledEnum"=w262) -> ()  [unwired: 2 in, 2 out]
                  }
                  frame False {
                    w263 = T3."Disabled and Grayed Out" ("禁用")
                    n172 = property on="GPIB Address_MPM" class="DigNum (严格)"("DisabledEnum"=T3."Enabled" ("禁用")) -> ()  [unwired: 2 in, 2 out]
                    n173 = property on="GPIB Address_MPM 2" class="DigNum (严格)"("DisabledEnum"=w263) -> ()  [unwired: 2 in, 2 out]
                    n174 = property on="LAN Port_MPM" class="DigNum (严格)"("DisabledEnum"=w263) -> ()  [unwired: 2 in, 2 out]
                    n175 = property on="LAN Port_MPM 2" class="DigNum (严格)"("DisabledEnum"=w263) -> ()  [unwired: 2 in, 2 out]
                    n176 = property on="IP Address_MPM 2" class="Str"("DisabledEnum"=w263) -> ()  [unwired: 2 in, 2 out]
                    n177 = property on="IP Address_MPM" class="Str"("DisabledEnum"=w263) -> ()  [unwired: 2 in, 2 out]
                  }
                }
              }
            }
          }
          event Panel Close? {
            n178 = event-data() -> ()  [unwired: 1 in, 4 out]
            n179 = event-data("Discard?"=TRUE ("放弃？")) -> ()  [unwired: 1 in, 1 out]
            "Boolean" <- FALSE
          }
        }
      }
    }
  }
  "Address Cluster out" <- w3
  "PowerMonitorType" <- w2
  n180 = global write "PowerMonitorType.vi" "PowerMonitorType"(w2) -> ()
  n181 = global write "PowerMonitorType.vi" "Product_MPM"(w1) -> ()
  n182 = call <vilib>:"General Error Handler.vi"("error in (no error)"=w6) -> ("error out"=→"错误输出":errorcluster)  [unwired: 10 in, 4 out]
